vi "Channel Array Size Error Test.vi"(8 "error in":errorcluster, 11 "NI 9422 test in":refnum<class "NI 9422 Test.lvclass">) -> (0 "error out":errorcluster, 3 "NI 9422 test out":refnum<class "NI 9422 Test.lvclass">)   [LabVIEW 2017, in "NI 9422 Test.lvclass"]
uses:
  NI 9422 Test.lvclass
  Module Test.lvclass
  Scripting/Modules/NI 9422/NI 9422.lvclass
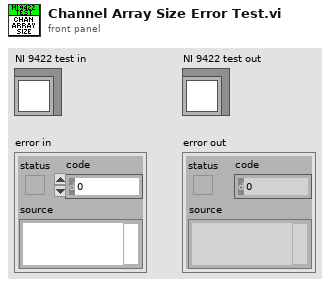
[diagram p1: front panel]
types:
  T1 = typedef "Scan Engine Scripting.lvlib/digital channel settings.ctl" = cluster{"name":string, "default value":bool}
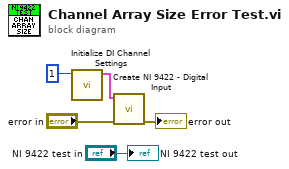
[diagram p0: block diagram]
diagram:
  n1 = call "Initialize DI Channel Settings.vi"("array size"=1) -> ("channel settings"=w1:T1[])  [unwired: 10 in]
  n2 = call "Create NI 9422 - Digital Input.vi"("error in"="error in", "channel settings"=w1) -> ("error out"=→"error out":errorcluster)  [unwired: 8 in, 1 out]
  "NI 9422 test out" <- "NI 9422 test in"
